vi "Configure Digital Pattern Repeat.vi"(8 "error in (no error)":errorcluster, 10 "Reapeat? (No)":bool, 11 "VISA resource name":refnum<visa-resource-name>) -> (0 "error out":errorcluster, 3 "VISA resource name out":refnum<visa-resource-name>)   [LabVIEW 2017, in "Keithley 3390.lvlib"]
doc: "Sets whether the digital pattern repeats or not."
uses:
  Keithley 3390.lvlib
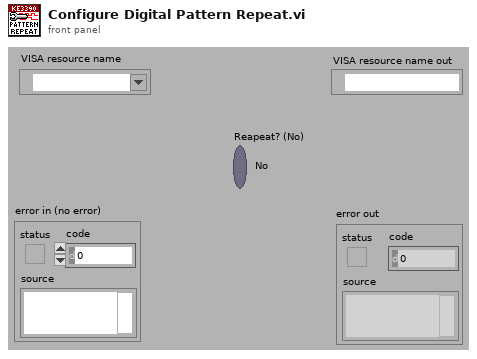
[diagram p1: front panel]
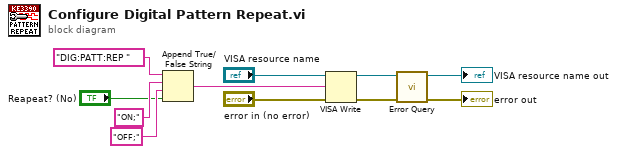
[diagram p0: block diagram]
diagram:
  n1 = Append True/False String(1:"Reapeat? (No)", 2:"OFF;" ("false string"), 3:"ON;" ("true string"), 4:"DIG:PATT:REP " ("command")) -> (0:w7:string)
  n2 = VISA Write(VISA resource name="VISA resource name", write buffer=w7, error in (no error)="error in (no error)") -> (VISA resource name out=w1:refnum<visa-resource-name>, error out=w2:errorcluster)  [unwired: 1 out]
  n3 = call "Error Query.vi"("error in (no error)"=w2, "VISA resource name"=w1) -> ("error out"=→"error out":errorcluster, "VISA resource name out"=→"VISA resource name out":refnum<visa-resource-name>)  [unwired: 6 in, 2 out]
